vi "remove zero.vi"() -> ()   [LabVIEW 2017]
panel:
  out "before substring":string
  in  "string":string
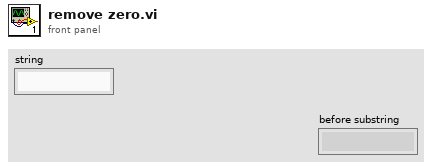
[diagram p1: front panel]
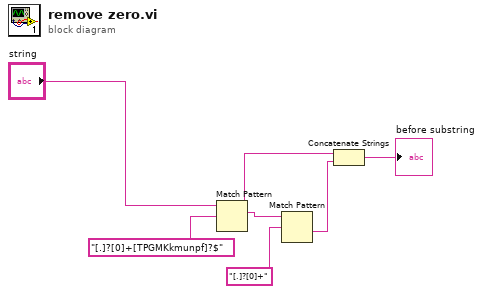
[diagram p0: block diagram]
diagram:
  n1 = Match Pattern(string="string", regular expression="[.]?[0]+[TPGMKkmunpf]?$") -> (before substring=w5:string, match substring=w4:string)  [unwired: 1 in, 2 out]
  n2 = Match Pattern(string=w4, regular expression="[.]?[0]+") -> (after substring=w1:string)  [unwired: 1 in, 3 out]
  n3 = Concatenate Strings(w5, w1) -> (→"before substring":string)
